vi "Set RowSpan.vi"(8 "error in (no error)":errorcluster, 10 "RowSpan":i32, 11 "Cell in":refnum<class "Cell.lvclass">) -> (0 "error out":errorcluster, 3 "Cell out":refnum<class "Cell.lvclass">)   [LabVIEW 2023, in "SourceGrid.lvlib" / "Cell.lvclass"]
uses:
  Cell.lvclass
  Cell.lvclass/Cell.ctl
  D:/git/Sourcegrid-LabVIEW/dll/SourceGrid.dll
  dll/SourceGrid.dll
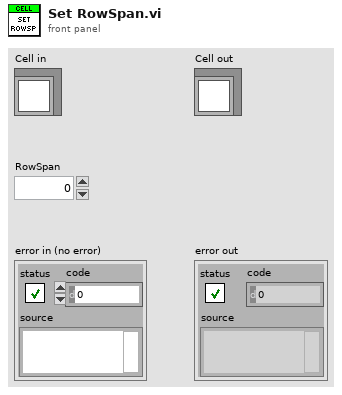
[diagram p1: front panel]
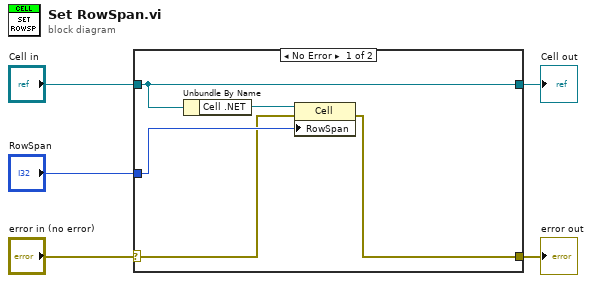
[diagram p0: block diagram]
diagram:
  n1 = case shown="No Error" "error in (no error)" {
    selector: "error in (no error)" -> [w7 w11]
    tunnel: [w6 w11] -> w4
    tunnel: [w10 w12] -> w2
    tunnel: "Cell in" -> [w10 w12]
    tunnel: "RowSpan" -> [w8 _]
    frame No Error {
      n2 = Unbundle By Name(w10) -> ("Cell .NET"=w9:refnum<k24>)
      n3 = property class="Cell"(reference=w9, error in=w7, "RowSpan"=w8) -> (error out=w6:errorcluster)  [unwired: 1 out]
    }
    frame Error {
    }
  }
  "error out" <- w4
  "Cell out" <- w2
